vi "WAVE get.vi"(1 "Command":string) -> (2 "OutPut":string)   [LabVIEW 2024]
panel:
  out "error out":errorcluster
  in  "error in (no error)":errorcluster
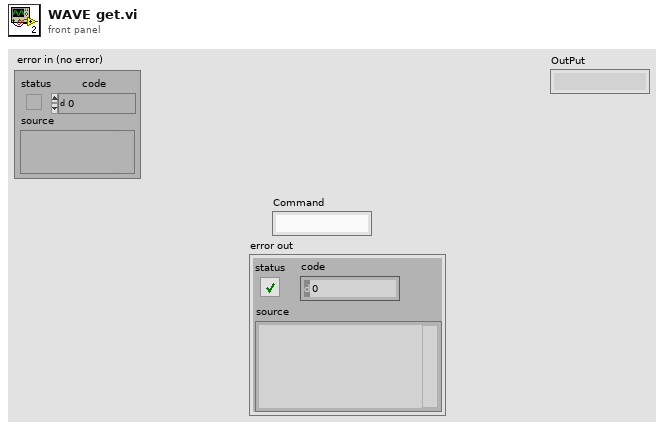
[diagram p1: front panel]
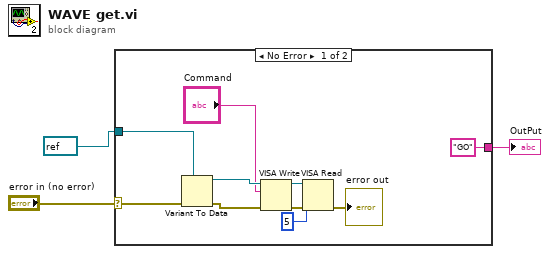
[diagram p0: block diagram]
diagram:
  n1 = case shown="No Error" "error in (no error)" {
    selector: "error in (no error)" -> [w8 _]
    tunnel: ["GO" ("read buffer") _] -> w2
    tunnel: refnum<visa-resource-name> refnum ("VISA resource name") -> [w4 _]
    frame No Error {
      n2 = Variant To Data(error in=w8, type=w4) -> (data=w13:refnum<visa-resource-name>, error out=w6:errorcluster)  [unwired: 1 in]
      n3 = VISA Write(VISA resource name=w13, write buffer="Command", error in (no error)=w6) -> (VISA resource name out=w12:refnum<visa-resource-name>, error out=w11:errorcluster)  [unwired: 1 out]
      n4 = VISA Read(VISA resource name=w12, byte count=u32 5, error in (no error)=w11) -> (error out=→"error out":errorcluster)  [unwired: 3 out]
    }
    frame Error {
    }
  }
  "OutPut" <- w2
